vi "CameraQueryAcquire.vi"(8 "error in (no error)":errorcluster, 11 "AndorSDK3 in":refnum<class "Andor3.lvclass">) -> (0 "error out":errorcluster, 1 "frames":u32, 2 "acquiring":bool, 3 "AndorSDK3 out":refnum<class "Andor3.lvclass">)   [LabVIEW 2010, in "Andor3.lvclass"]
doc: "Returns an array of camera communicated with by this SDK"
uses:
  Andor3.lvclass
  Andor3.lvclass/Andor3.ctl
  <userlib>/atcoreA/atcoreA.lvlib
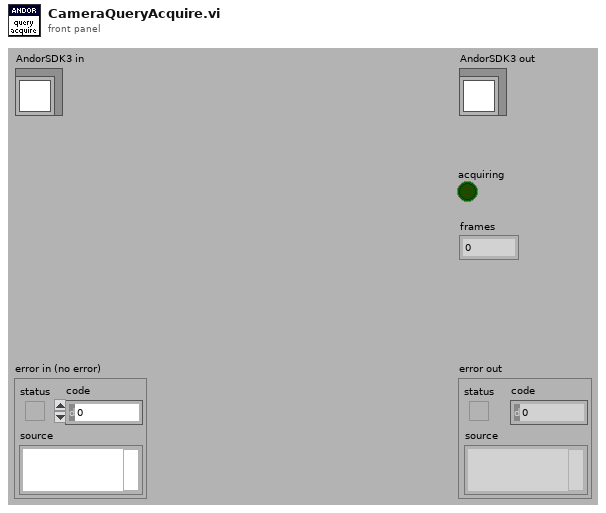
[diagram p1: front panel]
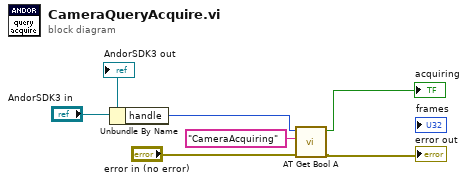
[diagram p0: block diagram]
diagram:
  n1 = Unbundle By Name("AndorSDK3 in") -> ("handle"=w3:i32)
  n2 = call <userlib>:"AT Get Bool A.vi"("error in (no error)"="error in (no error)", "Feature"="CameraAcquiring", "Hndl"=w3) -> ("error out"=→"error out":errorcluster, "Value"=→"acquiring":bool)  [unwired: 7 in]
  "AndorSDK3 out" <- "AndorSDK3 in"
